vi "Color Dialog.vi"(0 "Color in":u32) -> (4 "Color out":u32, 8 "Canceled?":bool)   [LabVIEW 2020, in "Filter (G3).xctl"]
uses:
  Filter (G3).xctl
panel:
  in  "Label color":u32(colorbox)
  out "exit signal":bool
  in  "Cancel":bool
  in  "OK":bool
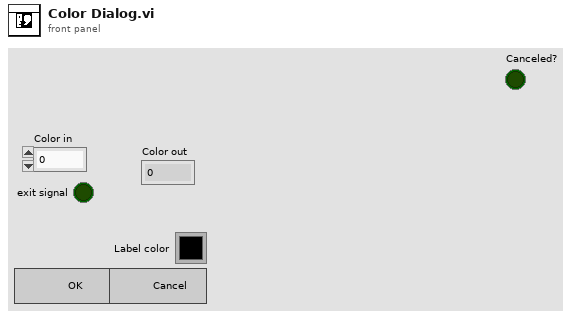
[diagram p1: front panel]
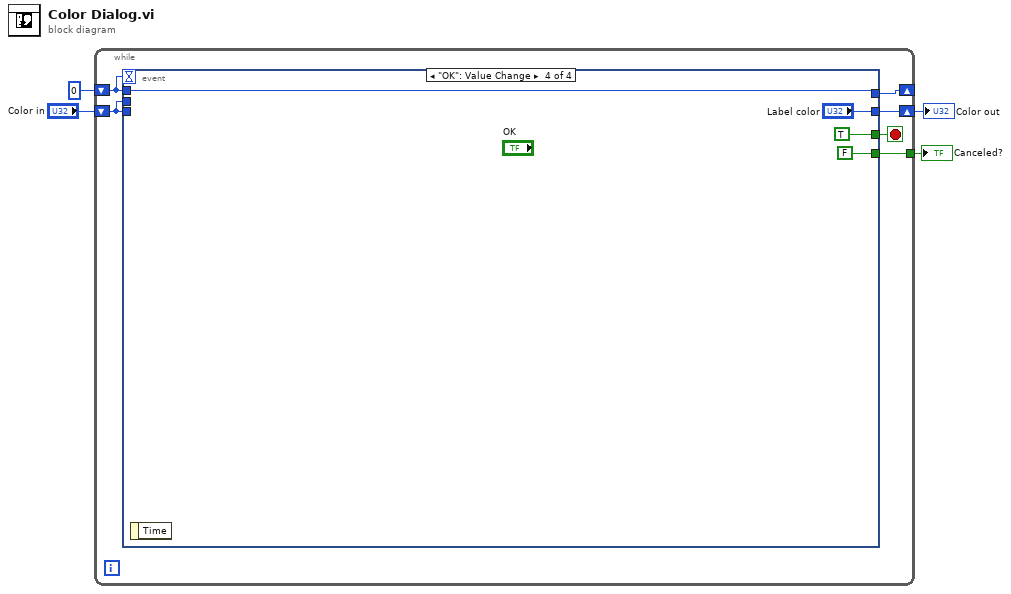
[diagram p0: block diagram]
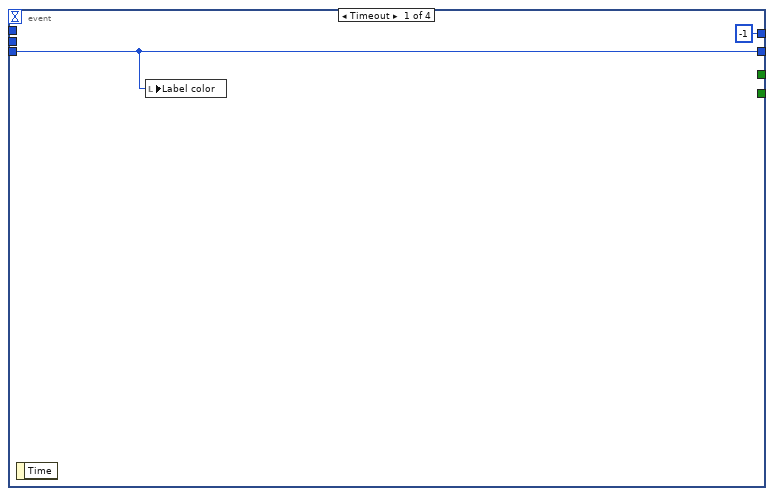
[diagram p2: hidden frame]
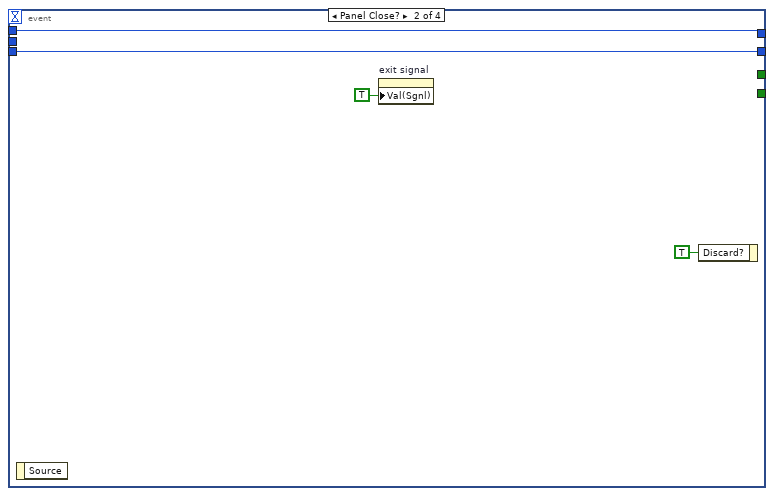
[diagram p3: hidden frame]
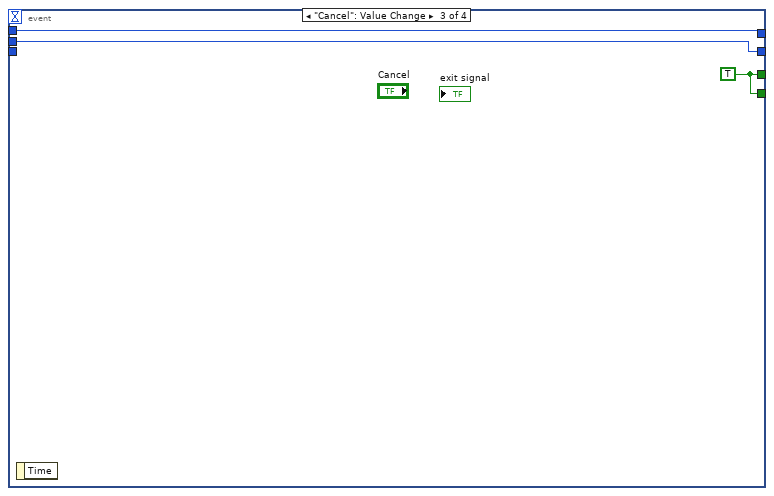
[diagram p4: hidden frame]
diagram:
  n1 = while {
    shift-right: [w10] -> _
    shift-left: 0 -> [w5]
    tunnel: [w7] -> w3
    shift-right: [w9] -> w2
    shift-left: "Color in" -> [w6]
    stop <- w8 stop-if-true
    n2 = event shown="[3] \"OK\": Value Change" {
      selector: _ -> [_ _ _ _]
      dyn-events: _ -> [_ _ _ _]
      timeout: w5 -> [_ _ _ _]
      tunnel: [-1 w16 w17 w21] -> w10
      tunnel: w6 -> [w11 w15 _ _]
      tunnel: [w11 w15 w18 "Label color"] -> w9
      tunnel: [_ _ w19 TRUE] -> w8
      tunnel: [_ _ w19 FALSE] -> w7
      tunnel: w6 -> [_ _ w18 _]
      tunnel: w5 -> [_ w16 w17 w21]
      event Timeout {
        n3 = event-data() -> ()  [unwired: 1 in, 1 out]
        n4 = local write "Label color"(w11) -> ()
      }
      event Panel Close? {
        n5 = event-data() -> ()  [unwired: 1 in, 1 out]
        n6 = property on="exit signal" class="Bool (strict)"("Val(Sgnl)"=TRUE ("Value (Signaling)")) -> ()  [unwired: 2 in, 2 out]
        n7 = event-data("Discard?"=TRUE) -> ()  [unwired: 1 in, 1 out]
      }
      event "Cancel": Value Change {
        w19 = TRUE
        n8 = event-data() -> ()  [unwired: 1 in, 1 out]
      }
      event "OK": Value Change {
        n9 = event-data() -> ()  [unwired: 1 in, 1 out]
      }
    }
  }
  "Canceled?" <- w3
  "Color out" <- w2
